vi "Write ID.vi"(8 "error in (no error)":errorcluster, 10 "ID":string, 11 "Guardian Died Recheck Msg in":refnum<class "Guardian Died Recheck Msg.lvclass">) -> (0 "error out":errorcluster, 3 "Guardian Died Recheck Msg out":refnum<class "Guardian Died Recheck Msg.lvclass">)   [LabVIEW 2026, in "TALOS.lvlib" / "Guardian.lvlib" / "Guardian Died Recheck Msg.lvclass"]
uses:
  Guardian Died Recheck Msg.lvclass
  Guardian Died Recheck Msg.lvclass/Guardian Died Recheck Msg.ctl
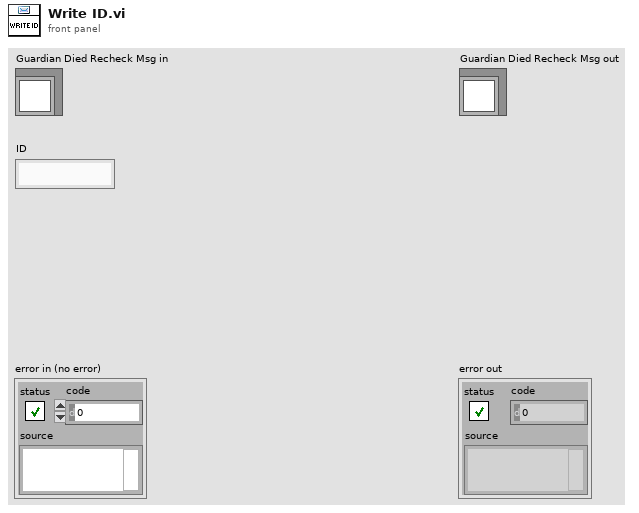
[diagram p1: front panel]
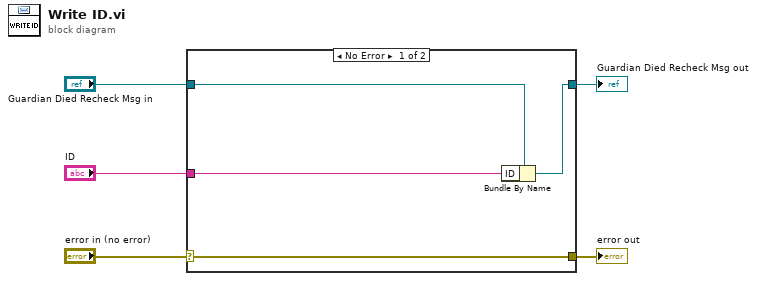
[diagram p0: block diagram]
diagram:
  n1 = case shown="No Error" "error in (no error)" {
    selector: "error in (no error)" -> [w9 w10]
    tunnel: [w9 w10] -> w4
    tunnel: [w7 w11] -> w2
    tunnel: "Guardian Died Recheck Msg in" -> [w8 w11]
    tunnel: "ID" -> [w6 _]
    frame No Error {
      n2 = Bundle By Name(cluster=w8, "ID"=w6) -> (w7:refnum<class "Guardian Died Recheck Msg.lvclass">)
    }
    frame Error {
    }
  }
  "error out" <- w4
  "Guardian Died Recheck Msg out" <- w2
